vi "Get Kasli IP.vi"(8 "error in (no error)":errorcluster, 11 "Kasli Listener in":refnum<class "Kasli Listener.lvclass">) -> (0 "error out":errorcluster, 3 "Kasli Listener out":refnum<class "Kasli Listener.lvclass">)   [LabVIEW 2020, in "CIRCUS_uServices.lvlib" / "Kasli Listener and Writer.lvlib" / "Kasli Listener.lvclass"]
uses:
  Kasli Listener.lvclass
  C:/Users/marco/Documents/GitHub_Lab/CIRCUS/TALOS/TALOS_PPL.lvlibp/Ancestor/Ancestor/Ancestor.lvclass
  C:/Users/marco/Documents/GitHub_Lab/CIRCUS/TALOS/TALOS_PPL.lvlibp/Internal uServices/System uServices/TCP Listener/TCP Listener/TCP Listener.lvclass
  TALOS/TALOS_PPL.lvlibp/Ancestor/Ancestor/Read ID.vi
  TALOS/TALOS_PPL.lvlibp
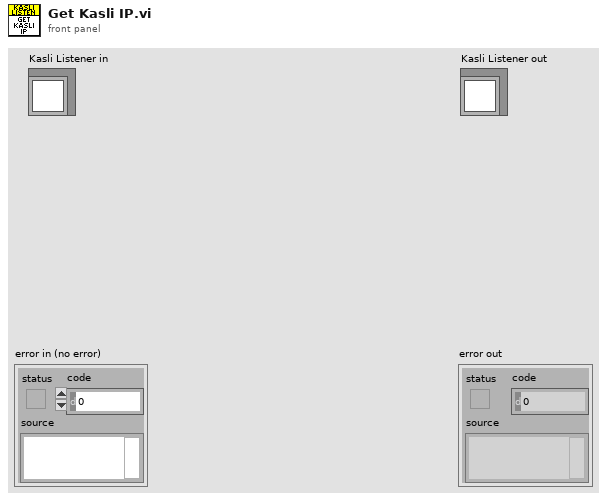
[diagram p1: front panel]
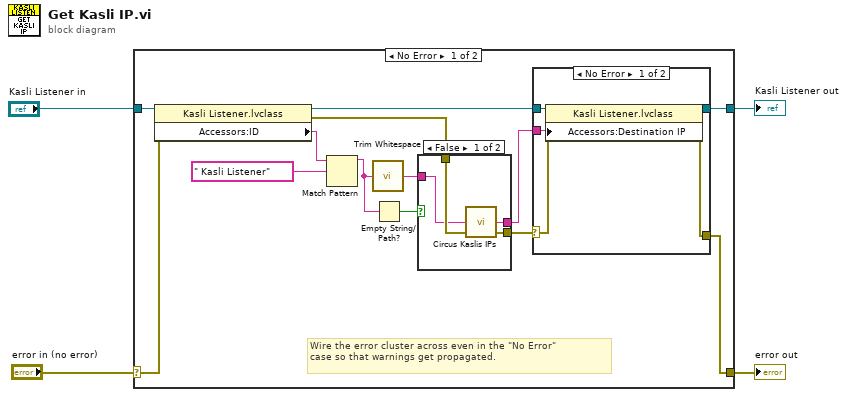
[diagram p0: block diagram]
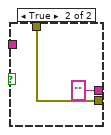
[diagram p3: hidden frame]
diagram:
  n1 = case shown="No Error" "error in (no error)" {
    selector: "error in (no error)" -> [w9 w32]
    tunnel: [w5 w32] -> w3
    tunnel: [w8 w31] -> w1
    tunnel: "Kasli Listener in" -> [w17 w31]
    frame No Error {
      # "Wire the error cluster across even in the \"No Error\"\ncase so that warnings get propagated."
      n2 = property class="Kasli Listener.lvclass"(reference=w17, error in=w9) -> (reference out=w16:refnum<class "Kasli Listener.lvclass">, error out=w10:errorcluster, "Accessors:ID"=w15:string)
      n3 = Match Pattern(string=w15, regular expression=" Kasli Listener") -> (before substring=w11:string)  [unwired: 1 in, 3 out]
      n4 = call <vilib>:"Trim Whitespace.vi"("string"=w11) -> ("trimmed string"=w12:string)  [unwired: 1 in]
      n5 = Empty String/Path?(string/path=w11) -> (empty?=w13:bool)
      n6 = case shown="False" w13 {
        tunnel: w12 -> [w25 _]
        tunnel: [w26 "" ("IP")] -> w7
        tunnel: [w27 w29] -> w6
        tunnel: w10 -> [w28 w29]
        frame False {
          n7 = call "Circus Kaslis IPs.vi"("error in (no error)"=w28, "ID"=w25) -> ("error out"=w27:errorcluster, "IP"=w26:string)  [unwired: 2 in]
        }
        frame True {
        }
      }
      n8 = case shown="No Error" w6 {
        selector: w6 -> [w22 w23]
        tunnel: w16 -> [w21 w24]
        tunnel: [w20 w24] -> w8
        tunnel: w7 -> [w19 _]
        tunnel: [w18 w23] -> w5
        frame No Error {
          n9 = property class="Kasli Listener.lvclass"(reference=w21, error in=w22, "Accessors:Destination IP"=w19) -> (reference out=w20:refnum<class "Kasli Listener.lvclass">, error out=w18:errorcluster)
        }
        frame Error {
        }
      }
    }
    frame Error {
    }
  }
  "error out" <- w3
  "Kasli Listener out" <- w1
